vi "Excel Write Data.vi"(8 "error in":errorcluster, 9 "Header Size":i32, 10 "Data":dbl[][](array[numeric]), 11 "_Worksheet In":refnum<k7>) -> (0 "error out":errorcluster, 3 "_Worksheet Out":refnum<k7>)   [LabVIEW 2012]
doc: "Writes data to Excel worksheet. Data must be in 1D row array. Header size is number of rows taken up by header lines."
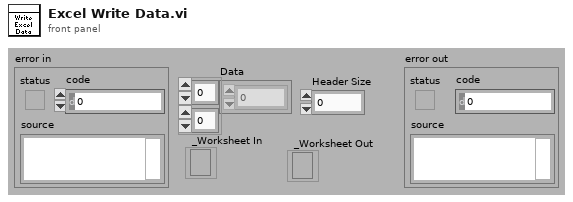
[diagram p1: front panel]
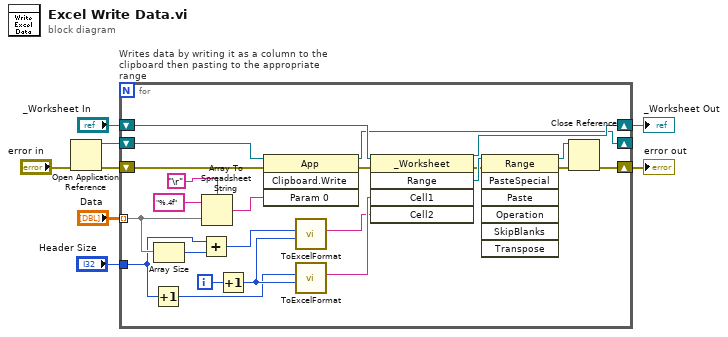
[diagram p0: block diagram]
diagram:
  n1 = Open Application Reference(8:"error in") -> (0:w2:errorcluster, 3:w1:refnum<vi>)  [unwired: 3 in]
  n2 = for "Writes data by writing it as a column to the clipboard then pasting to the appropriate range" {
    shift-right: [w30] -> w5
    shift-left: w2 -> [w14]
    shift-right: [w29] -> w4
    shift-left: "_Worksheet In" -> [w31]
    tunnel: "Data" -> [w17] mode=indexing
    shift-right: [w16] -> _
    shift-left: w1 -> [w15]
    tunnel: "Header Size" -> [w9]
    i -> [w22]
    n3 = Increment(x=w9) -> (x+1=w12:i32)
    n4 = Array Size(array=w17) -> (size(s)=w11:i32)
    n5 = Add(x=w9, y=w11) -> (x+y=w10:i32)
    n6 = Array To Spreadsheet String(delimiter (Tab)="\r", array=w17, 3:"%.4f" ("format string")) -> (spreadsheet string=w20:string)
    n7 = Increment(x=w22) -> (x+1=w21:i32)
    n8 = invoke class="App" method="Clipboard.Write"(reference=w15, error in=w14, "Param 0"=w20) -> (reference out=w16:refnum<vi>, error out=w13:errorcluster)  [unwired: 1 in, 2 out]
    n9 = call "ToExcelFormat.vi"("Column"=w21, "Row"=w10) -> ("Output String"=w23:string)  [unwired: 9 in]
    n10 = call "ToExcelFormat.vi"("Column"=w21, "Row"=w12) -> ("Output String"=w24:string)  [unwired: 9 in]
    n11 = invoke class="_Worksheet" method="Range"(reference=w31, error in=w13, "Cell1"=w24, "Cell2"=w23) -> (reference out=w29:refnum<k7>, error out=w26:errorcluster, "Range"=w28:refnum<k7>)  [unwired: 1 in, 2 out]
    n12 = invoke class="Range" method="PasteSpecial"(reference=w28, error in=w26) -> (reference out=w27:refnum<k7>, error out=w25:errorcluster)  [unwired: 5 in, 5 out]
    n13 = Close Reference(reference=w27, error in (no error)=w25) -> (error out=w30:errorcluster)
  }
  "error out" <- w5
  "_Worksheet Out" <- w4
